vi "automateRelayShortCircuit_IT6412w2110.vi"() -> ()   [LabVIEW 2023]
uses:
  IT64001/IT6400.lvlib
panel:
  in  "sign":bool=TRUE
  in  "loop index":i32
  out "error out 5":errorcluster
  in  "CV":bool
  in  "switchTime/s":i32=50
  in  "relay 2 (unshort)":bool
  out "Current through 330 ohm resistor/mA 6":cluster{"Y":dbl[], "Y":dbl[]}[](graph)
  out "Voltage across 330 ohm resistor 7":dbl[](graph)
  out "Voltage across 330 ohm resistor 8":dbl[](array[numeric])
  out "Current time":timestamp
  out "Voltage/V":cluster{"Y":dbl[], "Y":dbl[]}[](graph)
  out "Voltage":dbl[](graph)
  out "Voltage 2":dbl[](array[numeric])
  in  "Filename 4":path caption="Filename"
  in  "flag 2":bool
  out "error out 2":errorcluster
  in  "error in (no error) 4":errorcluster
  in  "VISA relay":refnum<visa-resource-name>="COM4"
  in  "VISA 2110 current":refnum<visa-resource-name>="USB0::0x05E6::0x2110::8017058::INSTR"
  in  "VISA 2110 voltage":refnum<visa-resource-name>="USB0::0x05E6::0x2110::8016020::INSTR"
  out "error out 4":errorcluster
  out "error out 3":errorcluster
  in  "Camera":bool
  out "Start time":timestamp
  in  "Countdown/s":i32=3
  out "Timer":dbl
  in  "error in (no error) 3":errorcluster
  in  "error in (no error) 2":errorcluster
  in  "stop 2":bool
  in  "Volt Limit (0 V)":dbl=9.0 min=0.0 max=15.0 format="%.3g"
  in  "Enable Volt Lim (T: Enable)":bool=TRUE
  in  "Curr Limit (0 A)":dbl=1.0 min=0.0 format="%.3g"
  in  "Enable Curr Lim (T: Enable)":bool=TRUE
  in  "Channel":i32=1 min=1 max=2
  in  "VOLT Range (0.0 v)":dbl=9.0 min=0.0 max=15.0 format="%.2g"
  in  "Enable OVP (T: Enable)":bool=TRUE
  in  "Reset":bool
  in  "Serial Configuration":T1={"Baud Rate"=9600, "Parity"=0, "Data Bits"=8, "Stop Bits"=10} {"Stop Bits" items=["1.0"=10, "1.5"=15, "2.0"=20]; "Data Bits" items=["7"=7, "8"=8]; "Parity" items=["None", "Odd", "Even", "Mark", "Space"]; "Baud Rate" items=["300"=300, "600"=600, "1200"=1200, "2400"=2400, "4800"=4800, "9600"=9600, "19200"=19200]}
  in  "Local/\nRemote":bool caption="Local/Remote"
  out "VISA resource name out":refnum<visa-resource-name>
  out "error out":errorcluster
  in  "error in (no error)":errorcluster
  in  "VISA resource name":refnum<visa-resource-name>="USB0::0x2EC7::0x6412::800624011767410027::INSTR"
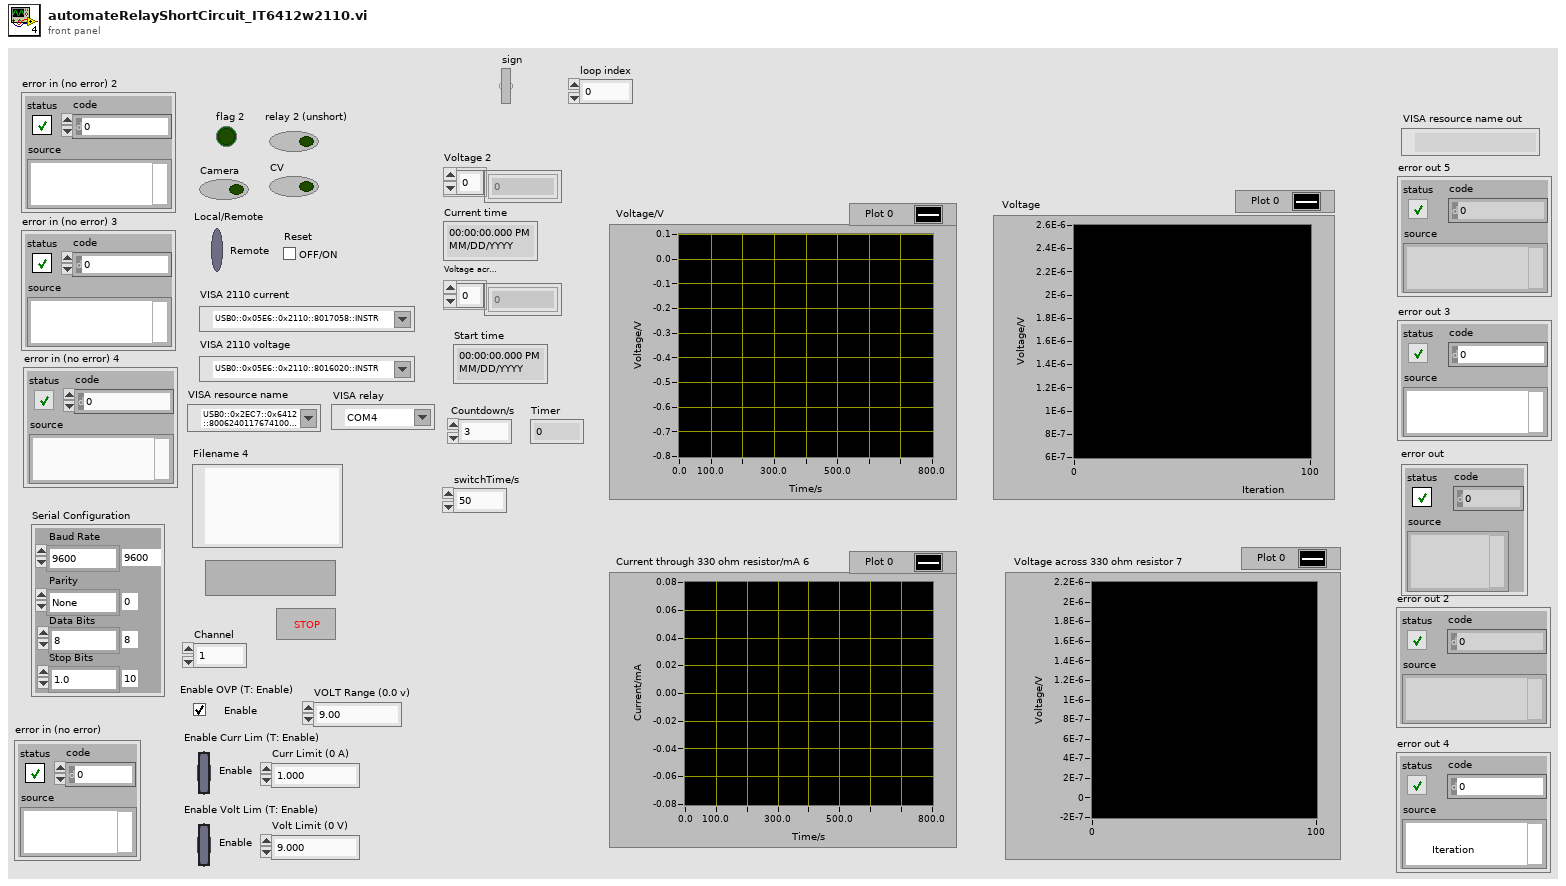
[diagram p1: front panel]
types:
  T1 = cluster{"Baud Rate":u32, "Parity":u16, "Data Bits":u16, "Stop Bits":u16}
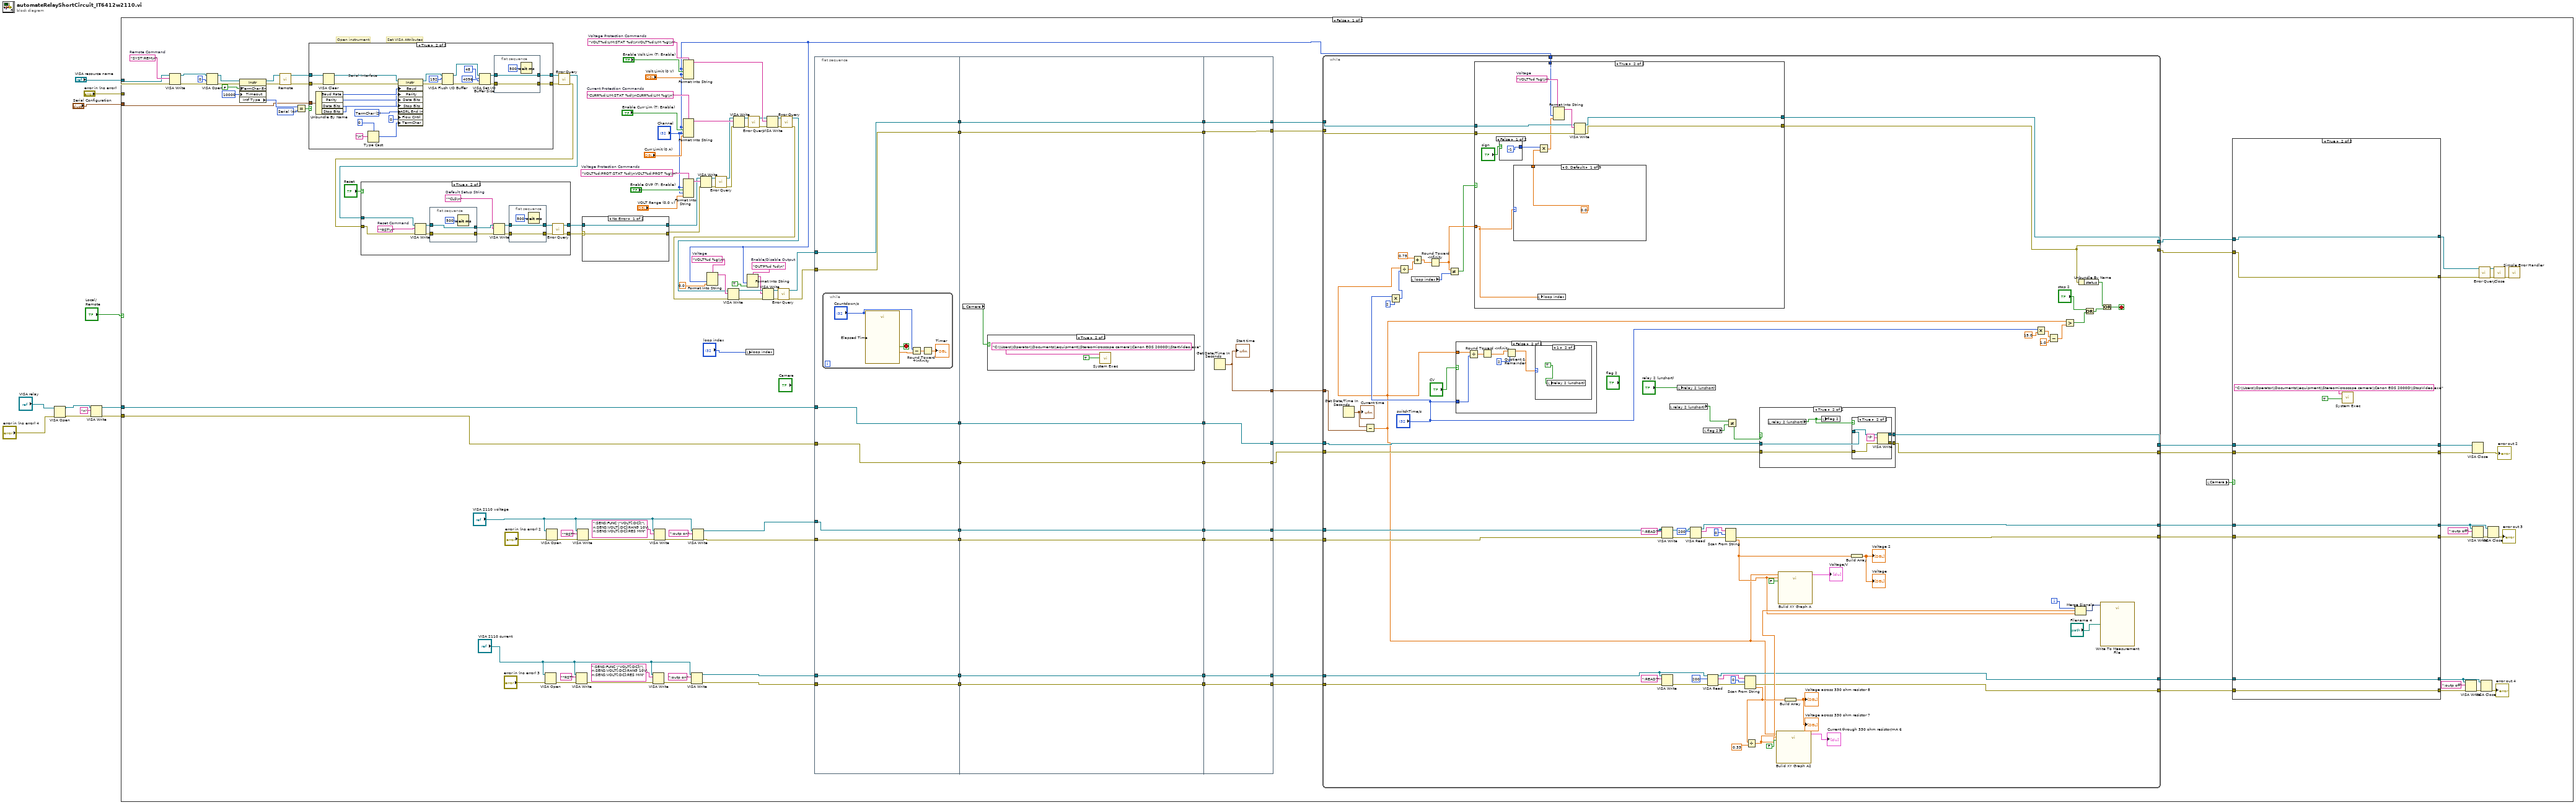
[diagram p0: block diagram]
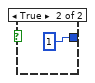
[diagram p5: hidden frame]
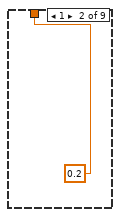
[diagram p6: hidden frame]
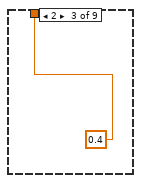
[diagram p7: hidden frame]
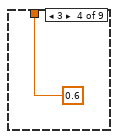
[diagram p8: hidden frame]
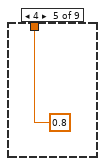
[diagram p9: hidden frame]
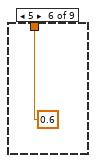
[diagram p10: hidden frame]
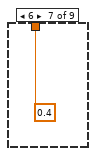
[diagram p11: hidden frame]
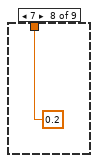
[diagram p12: hidden frame]
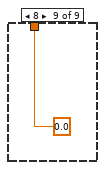
[diagram p13: hidden frame]
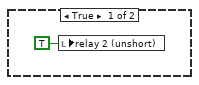
[diagram p14: hidden frame]
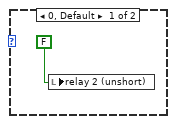
[diagram p15: hidden frame]
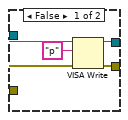
[diagram p17: hidden frame]
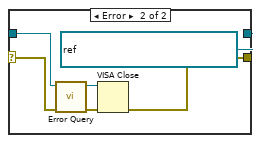
[diagram p18: hidden frame]
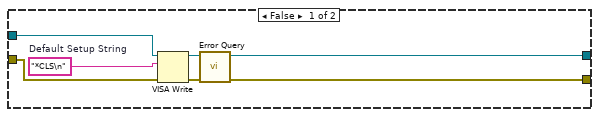
[diagram p19: hidden frame]
diagram:
  n1 = VISA Open(error in (no error)="error in (no error) 4", VISA resource name="VISA relay") -> (VISA resource name=w6:refnum<visa-resource-name>, error out=w7:errorcluster)  [unwired: 3 in]
  n2 = VISA Write(VISA resource name=w6, write buffer="n", error in (no error)=w7) -> (VISA resource name out=w1:refnum<visa-resource-name>, error out=w2:errorcluster)  [unwired: 1 out]
  n3 = case shown="False" "Local/\nRemote" {
    tunnel: "VISA resource name" -> [w45 w391]
    tunnel: "error in (no error)" -> [w44 w390]
    tunnel: "Serial Configuration" -> [w135 _]
    tunnel: w2 -> [w43 w386]
    tunnel: w1 -> [w42 w387]
    frame False {
      w20 = "VOLT%d %g\\n"  # Voltage
      w21 = "OUTP%d %d\n"  # Enable/Disable Output
      w115 = "VOLT%d:LIM:STAT %d\\nVOLT%d:LIM %g\\n"  # Voltage Protection Commands
      w123 = "CURR%d:LIM:STAT %d\\nCURR%d:LIM %g\\n"  # Current Protection Commands
      w129 = "VOLT%d:PROT:STAT %d\\nVOLT%d:PROT %g\\n"  # Voltage Protection Commands
      w148 = u16 4 items=["GPIB"=1, "VXI"=2, "GPIB-VXI"=3, "Serial"=4, "PXI"=5, "TCPIP"=6, "USB"=7] ("Interface Information:Interface Type")
      w150 = "SYST:REM\n"  # Remote Command
      # "Set VISA Attributes"
      # "Open instrument"
      n4 = VISA Write(VISA resource name=w45, write buffer=w150, error in (no error)=w44) -> (VISA resource name out=w134:refnum<visa-resource-name>, error out=w133:errorcluster)  [unwired: 1 out]
      n5 = VISA Open(access mode=u32 0, error in (no error)=w133, VISA resource name=w134) -> (VISA resource name=w146:refnum<visa-resource-name>, error out=w145:errorcluster)  [unwired: 2 in]
      n6 = property class="Instr"(reference=w146, error in=w145, "TermChar En"=FALSE, "Timeout"=u32 10000 ("General Settings:Timeout Value")) -> (reference out=w140:refnum<visa-resource-name>, error out=w139:errorcluster, "Intf Type"=w136:u16)
      n7 = call "Remote.vi"("error in (no error)"=w139, "VISA resource name"=w140) -> ("error out"=w141:errorcluster, "VISA resource name out"=w142:refnum<visa-resource-name>)  [unwired: 8 in]
      n8 = Equal?(x=w136, y=w148) -> (x = y?=w149:bool)
      n9 = case shown="True" w149 {
        tunnel: [w356 w360] -> w144
        tunnel: [w357 w359] -> w143
        tunnel: w142 -> [w356 w375]
        tunnel: w141 -> [w357 w374]
        tunnel: w135 -> [_ w358]
        frame False {
          # "EDIT: Remove interfaces not supported by your instrument."
          # "GPIB, TCP/IP, and USB Interface"
        }
        frame True {
          w369 = u16 2 items=["None", "LastBit", "TermChar"] ("Serial Settings:Serial End Mode for Reads")
          # "Serial Interface"
          n10 = Unbundle By Name(w358) -> ("Baud Rate"=w371:u32, "Parity"=w368:u16, "Data Bits"=w367:u16, "Stop Bits"=w370:u16)
          n11 = VISA Clear(VISA resource name=w375, error in (no error)=w374) -> (VISA resource name out=w373:refnum<visa-resource-name>, error out=w372:errorcluster)
          n12 = Type Cast(type=u8 0, x="\n" ("Line Feed Constant")) -> (*(type *) &x=w365:u8)
          n13 = property class="Instr"(reference=w373, error in=w372, "Baud"=w371, "Parity"=w368, "Data Bits"=w367, "Stop Bits"=w370, "ASRL End In"=w369, "Flow Cntrl"=0, "TermChar"=w365) -> (reference out=w381:refnum<visa-resource-name>, error out=w382:errorcluster)
          n14 = VISA Flush I/O Buffer(VISA resource name=w381, mask (16)=u16 192, error in (no error)=w382) -> (VISA resource name out=w364:refnum<visa-resource-name>, error out=w363:errorcluster)
          n15 = VISA Set I/O Buffer Size(VISA resource name=w364, mask (16)=u16 48, size (4096)=u32 4096 ("size (0)"), error in (no error)=w363) -> (VISA resource name out=w362:refnum<visa-resource-name>, error out=w361:errorcluster)
          n16 = flat-sequence {
            tunnel: w362 -> [w385]
            tunnel: w361 -> [w384]
            tunnel: [w385] -> w360
            tunnel: [w384] -> w359
            frame #0 {
              n17 = Wait (ms)(milliseconds to wait=500) -> ()  [unwired: 1 out]
            }
          }
        }
      }
      n18 = VISA Open(error in (no error)="error in (no error) 3", VISA resource name="VISA 2110 current") -> (error out=w92:errorcluster)  [unwired: 3 in, 1 out]
      n19 = VISA Open(error in (no error)="error in (no error) 2", VISA resource name="VISA 2110 voltage") -> (error out=w98:errorcluster)  [unwired: 3 in, 1 out]
      n20 = call "Error Query.vi"("error in (no error)"=w143, "VISA resource name"=w144) -> ("error out"=w46:errorcluster, "VISA resource name out"=w47:refnum<visa-resource-name>)  [unwired: 6 in, 2 out]
      n21 = case shown="True" "Reset" {
        tunnel: w47 -> [w334 w344]
        tunnel: w46 -> [w332 w343]
        tunnel: [w330 w337] -> w131
        tunnel: [w329 w336] -> w130
        frame False {
          w335 = "*CLS\n"  # Default Setup String
          n22 = VISA Write(VISA resource name=w334, write buffer=w335, error in (no error)=w332) -> (VISA resource name out=w333:refnum<visa-resource-name>, error out=w331:errorcluster)  [unwired: 1 out]
          n23 = call "Error Query.vi"("error in (no error)"=w331, "VISA resource name"=w333) -> ("error out"=w329:errorcluster, "VISA resource name out"=w330:refnum<visa-resource-name>)  [unwired: 6 in, 2 out]
        }
        frame True {
          w340 = "*CLS\n"  # Default Setup String
          w349 = "*RST\n"  # Reset Command
          n24 = VISA Write(VISA resource name=w344, write buffer=w349, error in (no error)=w343) -> (VISA resource name out=w348:refnum<visa-resource-name>, error out=w347:errorcluster)  [unwired: 1 out]
          n25 = flat-sequence {
            tunnel: w348 -> [w355]
            tunnel: [w355] -> w342
            tunnel: w347 -> [w353]
            tunnel: [w353] -> w341
            frame #0 {
              n26 = Wait (ms)(milliseconds to wait=500) -> ()  [unwired: 1 out]
            }
          }
          n27 = VISA Write(VISA resource name=w342, write buffer=w340, error in (no error)=w341) -> (VISA resource name out=w339:refnum<visa-resource-name>, error out=w338:errorcluster)  [unwired: 1 out]
          n28 = flat-sequence {
            tunnel: w339 -> [w352]
            tunnel: [w352] -> w346
            tunnel: [w350] -> w345
            tunnel: w338 -> [w350]
            frame #0 {
              n29 = Wait (ms)(milliseconds to wait=500) -> ()  [unwired: 1 out]
            }
          }
          n30 = call "Error Query.vi"("error in (no error)"=w345, "VISA resource name"=w346) -> ("error out"=w336:errorcluster, "VISA resource name out"=w337:refnum<visa-resource-name>)  [unwired: 6 in, 2 out]
        }
      }
      n31 = VISA Write(VISA resource name="VISA 2110 current", write buffer="*RST" ("数据"), error in (no error)=w92) -> (error out=w91:errorcluster)  [unwired: 2 out]
      n32 = VISA Write(VISA resource name="VISA 2110 voltage", write buffer="*RST" ("数据"), error in (no error)=w98) -> (error out=w97:errorcluster)  [unwired: 2 out]
      n33 = case shown="No Error" w130 {
        selector: w130 -> [w321 w324]
        tunnel: w131 -> [w322 w325]
        tunnel: [w322 refnum<visa-resource-name> "USB0::0x2EC7::0x6412::800624011767410027::INSTR" ("VISA resource name out")] -> w104
        tunnel: [w321 w323] -> w103
        frame No Error {
        }
        frame Error {
          n34 = call "Error Query.vi"("error in (no error)"=w324, "VISA resource name"=w325) -> ("error out"=w327:errorcluster, "VISA resource name out"=w326:refnum<visa-resource-name>)  [unwired: 6 in, 2 out]
          n35 = VISA Close(VISA resource name=w326, error in (no error)=w327) -> (error out=w323:errorcluster)
        }
      }
      n36 = VISA Write(VISA resource name="VISA 2110 current", write buffer=":SENS:FUNC \"VOLT[:DC]\"\n:SENS:VOLT[:DC]:RANG 10V\n:SENS:VOLT[:DC]:RES MIN" ("address string"), error in (no error)=w91) -> (error out=w90:errorcluster)  [unwired: 2 out]
      n37 = VISA Write(VISA resource name="VISA 2110 voltage", write buffer=":SENS:FUNC \"VOLT[:DC]\"\n:SENS:VOLT[:DC]:RANG 10V\n:SENS:VOLT[:DC]:RES MIN" ("address string"), error in (no error)=w97) -> (error out=w96:errorcluster)  [unwired: 2 out]
      n38 = Format Into String(format string=w115, "Channel", "Enable Volt Lim (T: Enable)", "Channel", "Volt Limit (0 V)") -> (resulting string=w112:string)  [unwired: 2 in, 1 out]
      n39 = Format Into String(format string=w123, "Channel", "Enable Curr Lim (T: Enable)", "Channel", "Curr Limit (0 A)") -> (resulting string=w120:string)  [unwired: 2 in, 1 out]
      n40 = Format Into String(format string=w129, "Channel", "Enable OVP (T: Enable)", "Channel", "VOLT Range (0.0 v)") -> (resulting string=w126:string)  [unwired: 2 in, 1 out]
      n41 = VISA Write(VISA resource name="VISA 2110 current", write buffer=":outp on" ("数据"), error in (no error)=w90) -> (VISA resource name out=w84:refnum<visa-resource-name>, error out=w83:errorcluster)  [unwired: 1 out]
      n42 = VISA Write(VISA resource name="VISA 2110 voltage", write buffer=":outp on" ("数据"), error in (no error)=w96) -> (VISA resource name out=w41:refnum<visa-resource-name>, error out=w37:errorcluster)  [unwired: 1 out]
      n43 = VISA Write(VISA resource name=w104, write buffer=w126, error in (no error)=w103) -> (VISA resource name out=w127:refnum<visa-resource-name>, error out=w128:errorcluster)  [unwired: 1 out]
      n44 = Format Into String(format string=w20, "Channel", 0.0 ("input 2")) -> (resulting string=w27:string)  [unwired: 2 in, 1 out]
      n45 = call "Error Query.vi"("error in (no error)"=w128, "VISA resource name"=w127) -> ("error out"=w116:errorcluster, "VISA resource name out"=w117:refnum<visa-resource-name>)  [unwired: 6 in, 2 out]
      n46 = VISA Write(VISA resource name=w117, write buffer=w120, error in (no error)=w116) -> (VISA resource name out=w121:refnum<visa-resource-name>, error out=w122:errorcluster)  [unwired: 1 out]
      n47 = local write "loop index"("loop index") -> ()
      n48 = Format Into String(format string=w21, "Channel", TRUE ("input 2")) -> (resulting string=w24:string)  [unwired: 2 in, 1 out]
      n49 = call "Error Query.vi"("error in (no error)"=w122, "VISA resource name"=w121) -> ("error out"=w108:errorcluster, "VISA resource name out"=w109:refnum<visa-resource-name>)  [unwired: 6 in, 2 out]
      n50 = VISA Write(VISA resource name=w109, write buffer=w112, error in (no error)=w108) -> (VISA resource name out=w113:refnum<visa-resource-name>, error out=w114:errorcluster)  [unwired: 1 out]
      n51 = call "Error Query.vi"("error in (no error)"=w114, "VISA resource name"=w113) -> ("error out"=w17:errorcluster, "VISA resource name out"=w16:refnum<visa-resource-name>)  [unwired: 6 in, 2 out]
      n52 = VISA Write(VISA resource name=w16, write buffer=w27, error in (no error)=w17) -> (VISA resource name out=w26:refnum<visa-resource-name>, error out=w25:errorcluster)  [unwired: 1 out]
      n53 = VISA Write(VISA resource name=w26, write buffer=w24, error in (no error)=w25) -> (VISA resource name out=w22:refnum<visa-resource-name>, error out=w23:errorcluster)  [unwired: 1 out]
      n54 = call "Error Query.vi"("error in (no error)"=w23, "VISA resource name"=w22) -> ("error out"=w14:errorcluster, "VISA resource name out"=w15:refnum<visa-resource-name>)  [unwired: 6 in, 2 out]
      n55 = flat-sequence {
        tunnel: w84 -> [w176]
        tunnel: [w176] -> w102
        tunnel: w83 -> [w175]
        tunnel: [w175] -> w101
        tunnel: [w174] -> w61
        tunnel: w15 -> [w174]
        tunnel: w14 -> [w173]
        tunnel: [w173] -> w58
        tunnel: w43 -> [w169]
        tunnel: w42 -> [w170]
        tunnel: w41 -> [w172]
        tunnel: [w172] -> w39
        tunnel: w37 -> [w171]
        tunnel: [w171] -> w35
        tunnel: [w170] -> w32
        tunnel: [w169] -> w29
        tunnel: [w189] -> w100
        tunnel: w102 -> [w189]
        tunnel: [w188] -> w99
        tunnel: w101 -> [w188]
        tunnel: [w187] -> w62
        tunnel: w61 -> [w187]
        tunnel: [w186] -> w59
        tunnel: w58 -> [w186]
        tunnel: [w185] -> w40
        tunnel: w39 -> [w185]
        tunnel: [w184] -> w36
        tunnel: w35 -> [w184]
        tunnel: [w183] -> w33
        tunnel: w32 -> [w183]
        tunnel: [w182] -> w30
        tunnel: w29 -> [w182]
        tunnel: [w201] -> w50
        tunnel: [w200] -> w52
        tunnel: w100 -> [w200]
        tunnel: [w199] -> w51
        tunnel: w99 -> [w199]
        tunnel: [w198] -> w60
        tunnel: w62 -> [w198]
        tunnel: [w197] -> w57
        tunnel: w59 -> [w197]
        tunnel: [w196] -> w38
        tunnel: w40 -> [w196]
        tunnel: [w195] -> w34
        tunnel: w36 -> [w195]
        tunnel: w33 -> [w194]
        tunnel: [w194] -> w31
        tunnel: [w193] -> w28
        tunnel: w30 -> [w193]
        frame #0 {
          n56 = while {
            stop <- w179 stop-if-true
            n57 = call "Elapsed Time"("Time Target (s)"="Countdown/s") -> ("Elapsed Time (s)"=w181:dbl, "Time has Elapsed"=w179:bool)  [unwired: 11 in, 6 out]
            n58 = Subtract(x="Countdown/s", y=w181) -> (x-y=w178:dbl)
            n59 = Round Toward +Infinity(x=w178) -> (ceil(x): smallest int >= x=→"Timer":dbl)
          }
        }
        frame #1 {
          n60 = local read "Camera"() -> (w190:bool)
          n61 = case shown="True" w190 {
            frame False {
            }
            frame True {
              n62 = call <vilib>:"System Exec.vi"("wait until completion? (T)"=TRUE, "command line"="C:\\Users\\Operator\\Documents\\equipment\\Stereomicroscope camera\\Canon EOS 2000D\\StartVideo.exe") -> ()  [unwired: 6 in, 4 out]
            }
          }
        }
        frame #2 {
          n63 = Get Date/Time In Seconds() -> (seconds since 1Jan1904=w201:timestamp)
          "Start time" <- w201
        }
      }
      n64 = while {
        tunnel: "Channel" -> [w263]
        tunnel: w60 -> [w267]
        tunnel: w57 -> [w266]
        tunnel: [w209] -> w64
        tunnel: [w210] -> w66
        tunnel: [w232] -> w56
        tunnel: [w231] -> w55
        tunnel: [w230] -> w54
        tunnel: [w229] -> w53
        tunnel: w52 -> [w227]
        tunnel: w51 -> [w226]
        tunnel: w50 -> [w225]
        tunnel: w38 -> [w224]
        tunnel: w34 -> [w223]
        tunnel: [w222] -> w49
        tunnel: [w221] -> w48
        tunnel: w31 -> [w220]
        tunnel: w28 -> [w219]
        i -> [w228]
        stop <- w268 stop-if-true
        n65 = Get Date/Time In Seconds() -> (seconds since 1Jan1904=w243:timestamp)
        "Current time" <- w243
        n66 = Subtract(x=w243, y=w225) -> (x-y=w208:dbl)
        n67 = Multiply(x="switchTime/s", y=2) -> (x*y=w265:i32)
        n68 = Divide(x=w208, y=w265) -> (x/y=w207:dbl)
        n69 = local read "loop index"() -> (w204:i32)
        n70 = Add(x=0.75, y=w207) -> (x+y=w205:dbl)
        n71 = Round Toward -Infinity(1:w205) -> (0:w203:dbl)
        n72 = Not Equal?(x=w203, y=w204) -> (x != y?=w202:bool)
        n73 = case shown="False" "CV" {
          tunnel: w208 -> [_ w298]
          tunnel: "switchTime/s" -> [_ w296]
          frame True {
            n74 = local write "relay 2 (unshort)"(TRUE ("relay 2 (unshort)")) -> ()
          }
          frame False {
            n75 = Divide(x=w298, y=w296) -> (x/y=w301:dbl)
            n76 = Round Toward -Infinity(1:w301) -> (0:w300:dbl)
            n77 = Quotient & Remainder(x=w300, y=2) -> (x-y*floor(x/y)=w297:dbl)  [unwired: 1 out]
            n78 = case shown="1" w297 {
              frame 0, Default {
                n79 = local write "relay 2 (unshort)"(FALSE) -> ()
              }
              frame 1 {
                n80 = local write "relay 2 (unshort)"(TRUE) -> ()
              }
            }
          }
        }
        n81 = case shown="True" w202 {
          tunnel: w267 -> [w271 w281]
          tunnel: w266 -> [w270 w280]
          tunnel: w263 -> [_ w279]
          tunnel: [w271 w278] -> w210
          tunnel: [w270 w277] -> w209
          tunnel: w203 -> [_ w276]
          frame False {
          }
          frame True {
            w282 = "VOLT%d %g\\n"  # Voltage
            n82 = case shown="False" "sign" {
              tunnel: [-1 1 ("sign")] -> w272
              frame False {
              }
              frame True {
              }
            }
            n83 = case shown="0, Default" w276 {
              tunnel: [0.0 0.2 0.4 0.6 0.8 0.6 0.4 0.2 0.0] -> w275
              frame 0, Default {
              }
              frame 1 {
              }
              frame 2 {
              }
              frame 3 {
              }
              frame 4 {
              }
              frame 5 {
              }
              frame 6 {
              }
              frame 7 {
              }
              frame 8 {
              }
            }
            n84 = local write "loop index"(w276) -> ()
            n85 = Multiply(x=w272, y=w275) -> (x*y=w274:dbl)
            n86 = Format Into String(format string=w282, w279, w274) -> (resulting string=w283:string)  [unwired: 2 in, 1 out]
            n87 = VISA Write(VISA resource name=w281, write buffer=w283, error in (no error)=w280) -> (VISA resource name out=w278:refnum<visa-resource-name>, error out=w277:errorcluster)  [unwired: 1 out]
          }
        }
        n88 = VISA Write(VISA resource name=w227, write buffer=":READ?" ("数据"), error in (no error)=w226) -> (error out=w247:errorcluster)  [unwired: 2 out]
        n89 = VISA Write(VISA resource name=w224, write buffer=":READ?" ("数据"), error in (no error)=w223) -> (error out=w256:errorcluster)  [unwired: 2 out]
        n90 = local read "relay 2 (unshort)"() -> (w234:bool)
        n91 = local write "relay 2 (unshort)"("relay 2 (unshort)") -> ()
        n92 = VISA Read(VISA resource name=w224, byte count=200 ("字节总数"), error in (no error)=w256) -> (VISA resource name out=w230:refnum<visa-resource-name>, read buffer=w258:string, error out=w257:errorcluster)  [unwired: 1 out]
        n93 = local read "flag 2"() -> (w262:bool)
        n94 = VISA Read(VISA resource name=w227, byte count=200 ("字节总数"), error in (no error)=w247) -> (VISA resource name out=w232:refnum<visa-resource-name>, read buffer=w249:string, error out=w248:errorcluster)  [unwired: 1 out]
        n95 = Scan From String(input string=w258, initial scan location=u32 0 ("初始扫描位置"), error in=w257) -> (error out=w229:errorcluster, output 1=w236:dbl)  [unwired: 2 in, 2 out]
        n96 = Not Equal?(x=w234, y=w262) -> (x != y?=w261:bool)
        n97 = Scan From String(input string=w249, initial scan location=u32 0 ("初始扫描位置"), error in=w248) -> (error out=w231:errorcluster, output 1=w238:dbl)  [unwired: 2 in, 2 out]
        n98 = Divide(x=w238, y=0.33) -> (x/y=w237:dbl)
        n99 = case shown="True" w261 {
          tunnel: w219 -> [w305 w307]
          tunnel: [w304 w310] -> w222
          tunnel: [w305 w309] -> w221
          tunnel: w220 -> [w304 w308]
          frame False {
          }
          frame True {
            n100 = local read "relay 2 (unshort)"() -> (w306:bool)
            n101 = local write "flag 2"(w306) -> ()
            n102 = case shown="True" w306 {
              tunnel: w308 -> [w312 w320]
              tunnel: w307 -> [w311 w318]
              tunnel: [w314 w317] -> w310
              tunnel: [w313 w316] -> w309
              frame False {
                n103 = VISA Write(VISA resource name=w312, write buffer="p", error in (no error)=w311) -> (VISA resource name out=w314:refnum<visa-resource-name>, error out=w313:errorcluster)  [unwired: 1 out]
              }
              frame True {
                n104 = VISA Write(VISA resource name=w320, write buffer="f", error in (no error)=w318) -> (VISA resource name out=w317:refnum<visa-resource-name>, error out=w316:errorcluster)  [unwired: 1 out]
              }
            }
          }
        }
        n105 = call "Bulid XY Graph A2"("Reset"=FALSE, "Y Input"=w237, "X Input"=w208) -> ("XY Graph"=→"Current through 330 ohm resistor/mA 6":cluster{"X":dbl[], "Y":dbl[]}[])  [unwired: 7 in, 1 out]
        n106 = call "Bulid XY Graph A"("Reset"=FALSE, "Y Input"=w236, "X Input"=w208) -> ("XY Graph"=→"Voltage/V":cluster{"X":dbl[], "Y":dbl[]}[])  [unwired: 7 in, 1 out]
        n107 = Build Array(w238) -> (→"Voltage across 330 ohm resistor 8" →"Voltage across 330 ohm resistor 7":dbl[])
        n108 = Build Array(w236) -> (→"Voltage 2" →"Voltage":dbl[])
        n109 = Multiply(x="switchTime/s", y=15.0) -> (x*y=w214:dbl)
        n110 = Subtract(x=w214, y=1.0) -> (x-y=w212:dbl)
        n111 = Greater?(x=w208, y=w212) -> (0:w217:bool)
        n112 = Merge Signals(w228, w237, w236) -> (w260:dynamicdata)
        n113 = Unbundle By Name(w209) -> ("status"=w269:bool)
        n114 = Or(x="stop 2", y=w217) -> (x .or. y?=w216:bool)
        n115 = call "Write To Measurement File"("Signals"=w260, "Filename"="Filename 4") -> ()  [unwired: 15 in, 3 out]
        n116 = Or(x=w269, y=w216) -> (x .or. y?=w268:bool)
      }
      n117 = local read "Camera"() -> (w76:bool)
      n118 = case shown="True" w76 {
        tunnel: [w158 w166] -> w75
        tunnel: w54 -> [w158 w166]
        tunnel: [w157 w165] -> w74
        tunnel: w53 -> [w157 w165]
        tunnel: [w156 w164] -> w73
        tunnel: w56 -> [w156 w164]
        tunnel: [w155 w163] -> w72
        tunnel: w55 -> [w155 w163]
        tunnel: w49 -> [w152 w162]
        tunnel: [w152 w162] -> w68
        tunnel: w48 -> [w151 w161]
        tunnel: [w151 w161] -> w67
        tunnel: w66 -> [w154 w160]
        tunnel: [w154 w160] -> w65
        tunnel: w64 -> [w153 w159]
        tunnel: [w153 w159] -> w63
        frame False {
        }
        frame True {
          n119 = call <vilib>:"System Exec.vi"("wait until completion? (T)"=TRUE, "command line"="C:\\Users\\Operator\\Documents\\equipment\\Stereomicroscope camera\\Canon EOS 2000D\\StopVideo.exe") -> ()  [unwired: 6 in, 4 out]
        }
      }
      n120 = VISA Write(VISA resource name=w73, write buffer=":outp off" ("数据"), error in (no error)=w72) -> (error out=w78:errorcluster)  [unwired: 2 out]
      n121 = VISA Write(VISA resource name=w75, write buffer=":outp off" ("数据"), error in (no error)=w74) -> (error out=w81:errorcluster)  [unwired: 2 out]
      n122 = VISA Close(VISA resource name=w68, error in (no error)=w67) -> (error out=→"error out 2":errorcluster)
      n123 = call "Error Query.vi"("error in (no error)"=w63, "VISA resource name"=w65) -> ("error out"=w107:errorcluster, "VISA resource name out"=w106:refnum<visa-resource-name>)  [unwired: 6 in, 2 out]
      n124 = VISA Close(VISA resource name=w73, error in (no error)=w78) -> (error out=→"error out 4":errorcluster)
      n125 = VISA Close(VISA resource name=w75, error in (no error)=w81) -> (error out=→"error out 3":errorcluster)
      n126 = call "Close.vi"("error in (no error)"=w107, "VISA resource name"=w106) -> ("error out"=w105:errorcluster)  [unwired: 9 in]
      n127 = call <vilib>:"Simple Error Handler.vi"("error in (no error)"=w105) -> ()  [unwired: 4 in, 5 out]
    }
    frame True {
      w389 = "SYST:LOC\n"  # Local Command
      n128 = VISA Close(VISA resource name=w387, error in (no error)=w386) -> (error out=→"error out 5":errorcluster)
      n129 = VISA Write(VISA resource name=w391, write buffer=w389, error in (no error)=w390) -> (VISA resource name out=w393:refnum<visa-resource-name>, error out=w392:errorcluster)  [unwired: 1 out]
      n130 = call "Error Query.vi"("error in (no error)"=w392, "VISA resource name"=w393) -> ("error out"=→"error out":errorcluster, "VISA resource name out"=→"VISA resource name out":refnum<visa-resource-name>)  [unwired: 6 in, 2 out]
    }
  }
